vi "Copy Setting.vi"(0 "VISA resource name":refnum<visa-resource-name>, 1 "Copy Mode (2:Dump)":u32(ring)=2 items=["Plot", "Print", "Dump"], 5 "Plot (0:All)":u32(ring) items=["All", "Graticule And Data", "Data"], 7 "PlotScale(0:Left,Bottom,Right,Top)":u32(ring) items=["Left, Bottom, Right, Top", "P1, P2 Normal", "P1, P2 Graticule Base"], 9 "Plot Scale - Left (2000)":i32=2000 min=0 max=100000, 11 "error in (no error)":errorcluster, 12 "Plot Scale - Bottom (800)":i32=800 min=0 max=100000, 13 "Plot Scale - Right (9200)":i32=9200 min=0 max=100000, 14 "Plot Scale - Top (7208)":i32=7208 min=0 max=100000) -> (4 "VISA resource name out":refnum<visa-resource-name>, 15 "error out":errorcluster)   [LabVIEW 2017, in "Agilent 4194.lvlib"]
doc: "This function sets the data copy function and copy parameters."
uses:
  Agilent 4194.lvlib
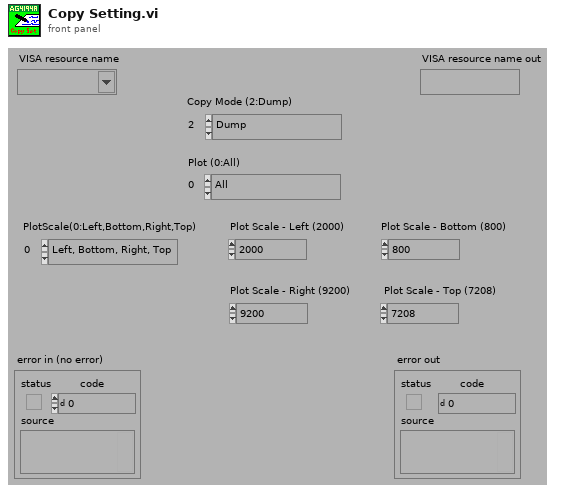
[diagram p1: front panel]
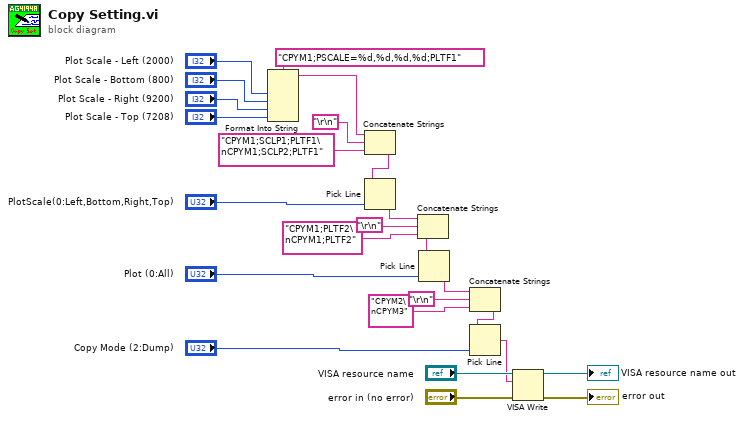
[diagram p0: block diagram]
diagram:
  n1 = Format Into String(format string="CPYM1;PSCALE=%d,%d,%d,%d;PLTF1", "Plot Scale - Left (2000)", "Plot Scale - Bottom (800)", "Plot Scale - Right (9200)", "Plot Scale - Top (7208)") -> (resulting string=w14:string)  [unwired: 2 in, 1 out]
  n2 = Concatenate Strings(w14, "\r\n", "CPYM1;SCLP1;PLTF1\nCPYM1;SCLP2;PLTF1" ("multi-line string")) -> (w16:string)
  n3 = Pick Line(multi-line string=w16, line index="PlotScale(0:Left,Bottom,Right,Top)") -> (output string=w13:string)  [unwired: 1 in]
  n4 = Concatenate Strings(w13, "\r\n", "CPYM1;PLTF2\nCPYM1;PLTF2") -> (w11:string)
  n5 = Pick Line(multi-line string=w11, line index="Plot (0:All)") -> (output string=w10:string)  [unwired: 1 in]
  n6 = Concatenate Strings(w10, "\r\n", "CPYM2\nCPYM3") -> (w6:string)
  n7 = Pick Line(multi-line string=w6, line index="Copy Mode (2:Dump)") -> (output string=w1:string)  [unwired: 1 in]
  n8 = VISA Write(VISA resource name="VISA resource name", write buffer=w1, error in (no error)="error in (no error)") -> (VISA resource name out=→"VISA resource name out":refnum<visa-resource-name>, error out=→"error out":errorcluster)  [unwired: 1 out]
